vi "get_sw_status.vi"(6 "error in (no error)":errorcluster, 9 "TCP Network Connection in":refnum<k5>) -> (0 "error out":errorcluster, 2 "Numeric":dbl, 3 "TCP Network Connection out":refnum<k5>)   [LabVIEW 2019]
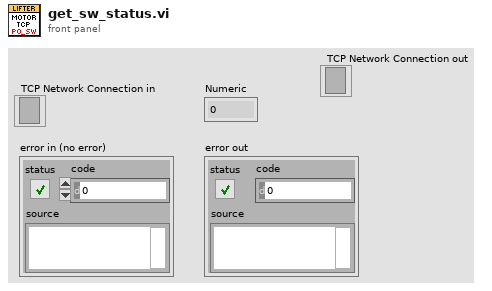
[diagram p1: front panel]
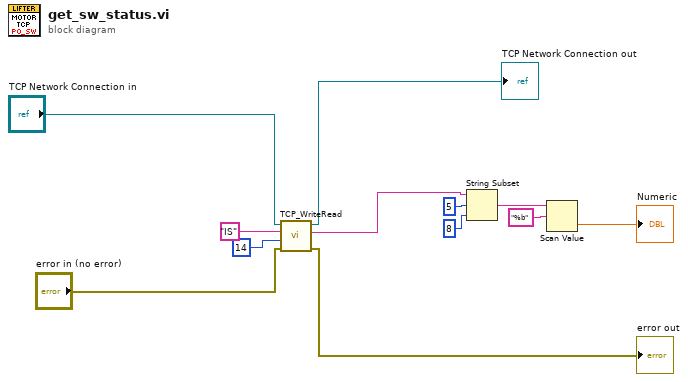
[diagram p0: block diagram]
diagram:
  n1 = call "TCP_WriteRead.vi"("error in"="error in (no error)", "bytes to read"=14, "Parameter 1"="IS" ("string"), "connection ID"="TCP Network Connection in") -> ("error out"=→"error out":errorcluster, "DataOut"=w1:string, "TCP Network Connection out"=→"TCP Network Connection out":refnum<k5>)  [unwired: 5 in]
  n2 = String Subset(string=w1, offset (0)=5, length (rest)=8 ("length (rest)")) -> (substring=w12:string)
  n3 = Scan Value(string=w12, format string="%b") -> (value=→"Numeric":dbl)  [unwired: 1 in, 1 out]
